vi "8-bit video export-Error handler.vi"(8 "error in (no error)":errorcluster, 11 "Stop":bool) -> ()   [LabVIEW 2017]
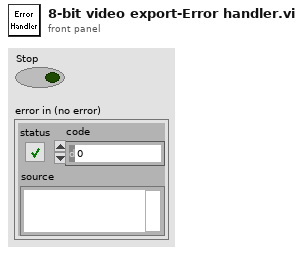
[diagram p1: front panel]
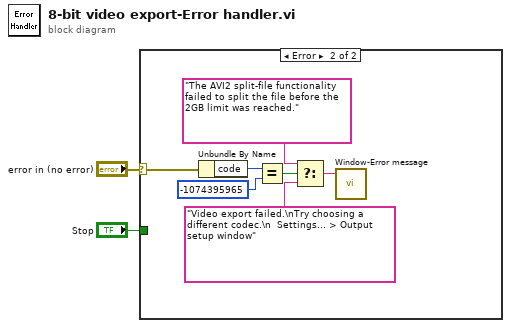
[diagram p0: block diagram]
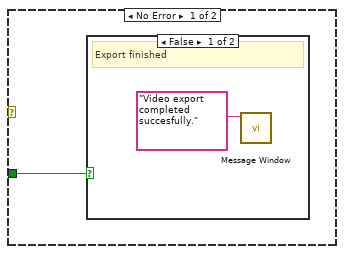
[diagram p2: hidden frame]
diagram:
  n1 = case shown="Error" "error in (no error)" {
    selector: "error in (no error)" -> [_ w11]
    tunnel: "Stop" -> [w3 _]
    frame No Error {
      n2 = case shown="False" w3 {
        frame False {
          # "Export finished"
          n3 = call "Message Window.vi"("Message string"="Video export completed succesfully.") -> ()  [unwired: 10 in, 1 out]
        }
        frame True {
          # "Stopped"
        }
      }
    }
    frame Error {
      n4 = Unbundle By Name(w11) -> ("code"=w10:i32)
      n5 = Equal?(x=w10, y=-1074395965 ("code")) -> (x = y?=w8:bool)
      n6 = Select(t="The AVI2 split-file functionality failed to split the file before the 2GB limit was reached.", s=w8, f="Video export failed.\nTry choosing a different codec.\n  Settings... > Output setup window") -> (s? t:f=w5:string)
      n7 = call "Window-Error message.vi"("Message"=w5) -> ()  [unwired: 10 in, 1 out]
    }
  }
